vi "Main.vi"(8 "error in (no error)":errorcluster, 11 "FMLazyEvaluationDemo":refnum<class "FMLazyEvaluationDemo.lvclass">) -> (0 "error out":errorcluster, 3 "FMLazyEvaluationDemo":refnum<class "FMLazyEvaluationDemo.lvclass">)   [LabVIEW 2020, in "FactoryMethod.lvlib" / "FactoryMethodLazyEvaluation.lvlib" / "FMLazyEvaluationDemo.lvclass"]
uses:
  FMLazyEvaluationDemo.lvclass
  CreatorA/CreatorA.lvclass
  E:/Francesco/GitHub/Design-Patterns-GoF_-_NI-LV/Creational/FactoryMethod/GoF_Example/FactoryMethodLazyEvaluation/Creator/Creator.lvclass
  CreatorB/CreatorB.lvclass
  Product/Product.lvclass
  Creator/Creator.lvclass
  Support/Class/ConsoleOutput.lvclass
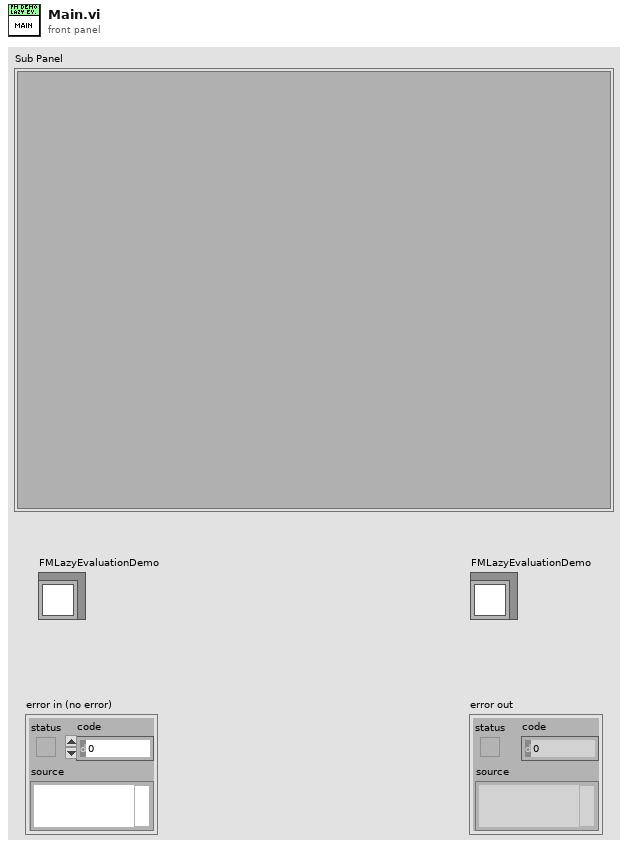
[diagram p1: front panel]
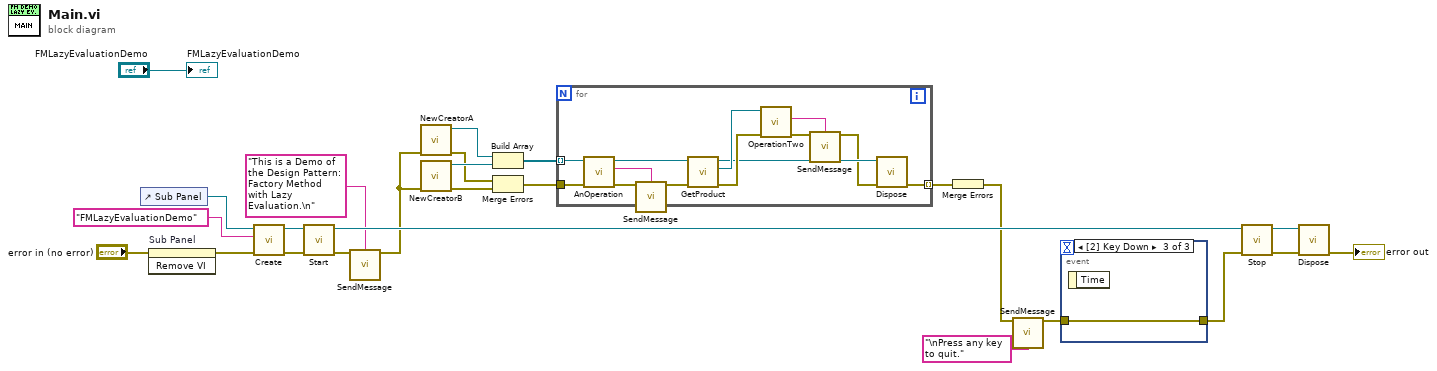
[diagram p0: block diagram]
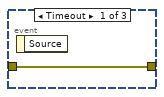
[diagram p2: hidden frame]
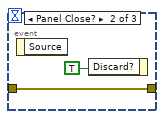
[diagram p3: hidden frame]
diagram:
  n1 = control-ref of="Sub Panel"() -> (w15:refnum<vi>)
  n2 = invoke on="Sub Panel" class="SubPnl" method="Remove VI"(error in="error in (no error)") -> (error out=w16:errorcluster)  [unwired: 2 in, 2 out]
  n3 = call "Create.vi"("error in (no error)"=w16, "LoggerName"="FMLazyEvaluationDemo", "SubPanelRef"=w15) -> ("error out"=w25:errorcluster, "ConsoleOutput out"=w24:refnum<class "ConsoleOutput.lvclass">)  [unwired: 7 in]
  n4 = call "Start.vi"("error in (no error)"=w25, "ConsoleOutput in"=w24) -> ("error out"=w17:errorcluster, "ConsoleOutput out"=w20:refnum<class "ConsoleOutput.lvclass">)  [unwired: 8 in]
  n5 = call "SendMessage.vi"("Message"="This is a Demo of the Design Pattern: Factory Method with Lazy Evaluation.\n" ("Data"), "error in (no error)"=w17) -> ("error out"=w8:errorcluster)  [unwired: 13 in]
  n6 = call "NewCreatorA.vi"("error in (no error)"=w8) -> ("error out"=w4:errorcluster, "CreatorA"=w7:refnum<class "CreatorA.lvclass">)  [unwired: 9 in]
  n7 = call "NewCreatorB.vi"("error in (no error)"=w8) -> ("error out"=w2:errorcluster, "CreatorB"=w6:refnum<class "CreatorB.lvclass">)  [unwired: 9 in]
  n8 = Build Array(w7, w6) -> (w5:refnum<class "Creator.lvclass">[])
  n9 = Merge Errors(w4, w2) -> (w3:errorcluster)
  n10 = for {
    tunnel: [w28] -> w9 mode=indexing
    tunnel: w5 -> [w27] mode=indexing
    tunnel: w3 -> [w26]
    n11 = call "AnOperation.vi"("error in (no error)"=w26, "Creator"=w27) -> ("error out"=w38:errorcluster, "ResultString"=w37:string, "Creator"=w35:refnum<class "Creator.lvclass">)  [unwired: 7 in]
    n12 = call "SendMessage.vi"("Message"=w37, "error in (no error)"=w38) -> ("error out"=w36:errorcluster)  [unwired: 13 in]
    n13 = call "GetProduct.vi"("error in"=w36, "Creator"=w35) -> ("error out"=w33:errorcluster, "Product"=w34:refnum<class "Product.lvclass">, "Creator"=w30:refnum<class "Creator.lvclass">)  [unwired: 7 in]
    n14 = call-dynamic "OperationTwo.vi"("error in (no error)"=w33, "Product in"=w34) -> ("error out"=w32:errorcluster, "ResultString"=w31:string)  [unwired: 7 in, 1 out]
    n15 = call "SendMessage.vi"("Message"=w31, "error in (no error)"=w32) -> ("error out"=w29:errorcluster)  [unwired: 13 in]
    n16 = call-dynamic "Dispose.vi"("error in (no error)"=w29, "IDisposable"=w30) -> ("error out"=w28:errorcluster)  [unwired: 9 in]
  }
  n17 = Merge Errors(w9) -> (w1:errorcluster)
  n18 = call "SendMessage.vi"("Message"="\nPress any key to quit." ("Data"), "error in (no error)"=w1) -> ("error out"=w13:errorcluster)  [unwired: 13 in]
  n19 = event shown="[2] Key Down" {
    selector: _ -> [_ _ _]
    dyn-events: _ -> [_ _ _]
    timeout: _ -> [_ _ _]
    tunnel: w13 -> [w39 w41 w42]
    tunnel: [w39 w41 w42] -> w18
    event Timeout {
      n20 = event-data() -> ()  [unwired: 1 in, 1 out]
    }
    event Panel Close? {
      n21 = event-data() -> ()  [unwired: 1 in, 1 out]
      n22 = event-data("Discard?"=TRUE) -> ()  [unwired: 1 in, 1 out]
    }
    event Key Down {
      n23 = event-data() -> ()  [unwired: 1 in, 1 out]
    }
  }
  n24 = call "Stop.vi"("error in (no error)"=w18, "ConsoleOutput in"=w20) -> ("error out"=w22:errorcluster, "ConsoleOutput out"=w21:refnum<class "ConsoleOutput.lvclass">)  [unwired: 8 in]
  n25 = call "Dispose.vi"("error in (no error)"=w22, "ConsoleOutput in"=w21) -> ("error out"=→"error out":errorcluster)  [unwired: 9 in]
  "FMLazyEvaluationDemo" <- "FMLazyEvaluationDemo"
